vi "Hold Boolean Signal.vi"(7 "reset":bool, 10 "width":fxp<+,5,5>, 11 "input signal":bool) -> (3 "output signal":bool)   [LabVIEW 2018]
doc: "Holds boolean signal <b>width</b> cycles"
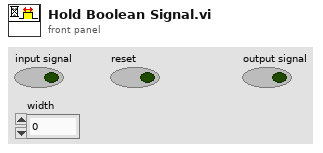
[diagram p1: front panel]
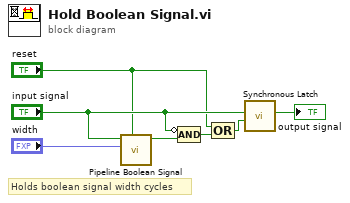
[diagram p0: block diagram]
diagram:
  # "Holds boolean signal width cycles"
  n1 = call "Pipeline Boolean Signal.vi"("reset"="reset", "delay"="width", "input signal"="input signal") -> ("output signal"=w5:bool)  [unwired: 8 in]
  n2 = Compound Arithmetic op=AND(invert "input signal", w5) -> (w2:bool)
  n3 = Compound Arithmetic op=OR("reset", w2) -> (w3:bool)
  n4 = call "Synchronous Latch.vi"("clear"=w3, "set"="input signal") -> ("out"=→"output signal":bool)  [unwired: 9 in]
